vi "Super Market Billing System edit 5.vi"() -> ()   [LabVIEW 2021]
uses:
  <vilib>/Utility/file.llb/Write Delimited Spreadsheet (string).vi
  <vilib>/regexp/Match Regular Expression.xnode
panel:
  in  "Tab Control":T1(tab)
  in  "2":bool caption="Blank Button"
  in  "1":bool caption="Blank Button"
  in  "Address":string
  in  "Telephone No:":string
  in  "Password":string
  in  "Email":string
  in  "Register Now":bool
  out "Horizontal Progress Bar 3":u8(slide) scale=0.0..100.0
  in  "adress":string
  out "Horizontal Progress Bar":u8(slide) scale=0.0..100.0
  in  "password":string
  in  "Email":string
  in  "OK Button":bool
  in  "Rise 5Kg":bool
  in  "Dal 1Kg":bool
  in  "Salt 400g":bool
  in  "Coconut Oil 1L":bool
  in  "Cilli Powder 100g":bool
  in  "Curry Powder 100g":bool
  in  "Turmeric Powder 50g":bool
  in  "Milk Powder 1kg":bool
  in  "Sugar  1kg":bool
  out "Rs.":dbl
  out "Rs.":dbl
  out "Rs.":dbl
  out "Rs.":dbl
  in  "Quantitiy":dbl min=0.0 format="%#.1f"
  out "Rs.":dbl
  in  "Quantitiy":dbl min=0.0 format="%#.1f"
  out "Rs":dbl
  in  "Quantitiy":dbl min=0.0 format="%#.1f"
  out "Rs.":dbl
  in  "Quantitiy":dbl min=0.0 format="%#.1f"
  in  "Quantitiy":dbl min=0.0 format="%#.1f"
  in  "Quantitiy":dbl min=0.0 format="%#.1f"
  in  "Quantitiy":dbl min=0.0 format="%#.1f"
  in  "Quantitiy":dbl min=0.0 format="%#.1f"
  in  "Tea 100g":bool
  in  "Quantitiy":dbl min=0.0 format="%#.1f"
  in  "Quantitiy":dbl min=0.0 format="%#.1f"
  out "Rs.":dbl
  out "Rs.":dbl
  out "Rs.":dbl
  out "Rs.":dbl
  out "Rs.":dbl
  out "Rs.":dbl
  out "Rs.":dbl
  out "Rs. 5":dbl
  out "Rs. 6":dbl
  out "Rs.":dbl
  out "Rs.":dbl
  out "Rs.":dbl
  out "Rs.":dbl
  out "Discount   Rs.":dbl format="%#.2f"
  in  "kg":dbl min=0.0 format="%#.3f"
  in  "Papaya":bool
  in  "kg":dbl min=0.0 format="%#.3f"
  in  "Graps":bool
  in  "kg":dbl min=0.0 format="%#.3f"
  in  "Orange":bool
  in  "kg":dbl min=0.0 format="%#.3f"
  in  "Apple":bool
  in  "kg":dbl min=0.0 format="%#.3f"
  in  "Banana":bool
  out "Bill   Rs.":dbl format="%#.2f"
  out "Discount percentage":string
  out "Total Bill   Rs.":dbl format="%#.2f"
  in  "kg":dbl min=0.0 format="%#.3f"
  in  "Cabege":bool
  in  "kg":dbl min=0.0 format="%#.3f"
  in  "Bringle":bool
  in  "kg":dbl min=0.0 format="%#.3f"
  in  "Beans":bool
  in  "kg":dbl min=0.0 format="%#.3f"
  in  "Leeks":bool
  in  "kg":dbl min=0.0 format="%#.3f"
  in  "Carrot":bool
  in  "stop":bool
  in  "stop 2":bool
  out "Your Bill Details":string
  in  "stop 3":bool
  # "WELCOME TO A SUPER MARCKET...."
  # "Register Here"
  # "Logging Here"
  # "Price per 1kg (Rs.)"
  # "Quantities(kg)"
  # "Price  (Rs.)"
  # "Quantities"
  # "Vegetables"
  # "Product List"
  # "Fruits"
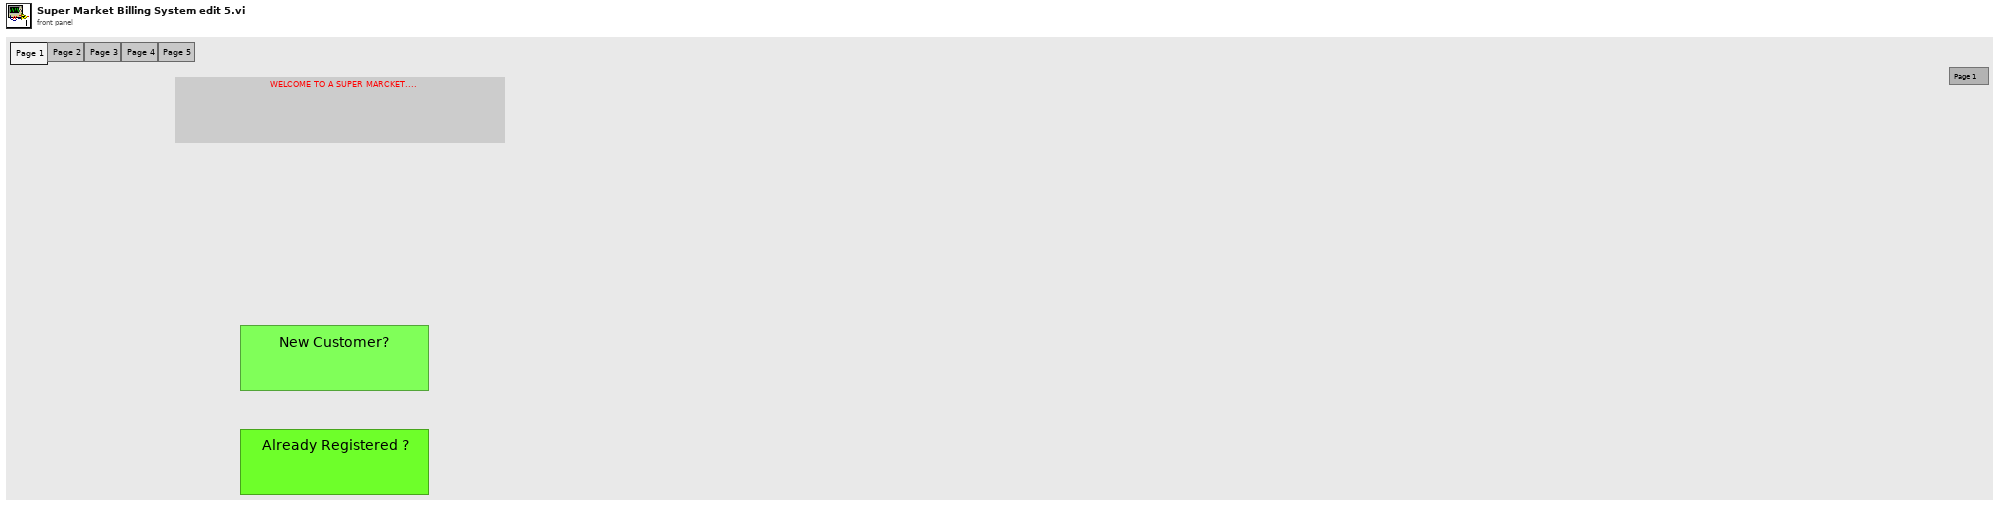
[diagram p1: front panel]
types:
  T1 = enum32{"Page 1", "Page 2", "Page 3", "Page 4", "Page 5"}
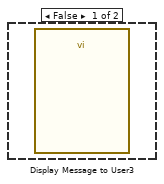
[diagram p2: hidden frame]
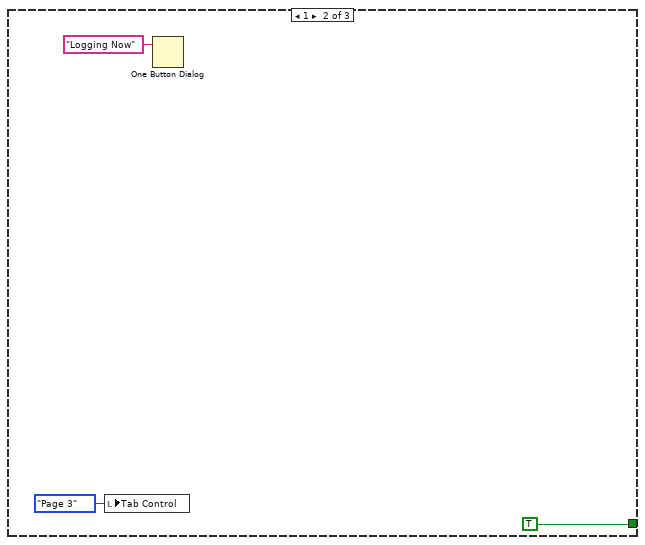
[diagram p4: hidden frame]
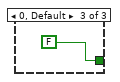
[diagram p5: hidden frame]
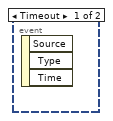
[diagram p6: hidden frame]
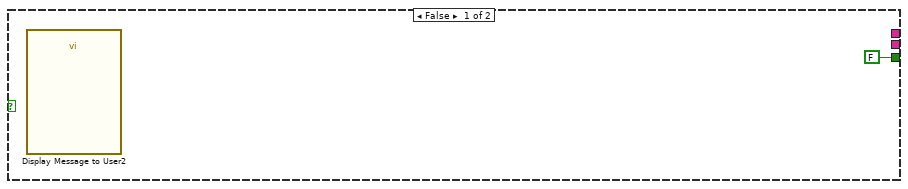
[diagram p7: hidden frame]
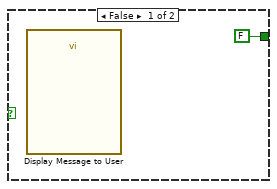
[diagram p8: hidden frame]
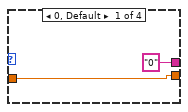
[diagram p9: hidden frame]
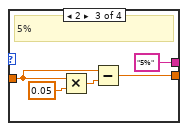
[diagram p10: hidden frame]
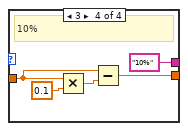
[diagram p11: hidden frame]
diagram:
  n1 = while {
    stop <- FALSE stop-if-true
    n2 = flat-sequence {
      tunnel: [w95] -> w51
      tunnel: [w89] -> w6
      tunnel: w51 -> [w448]
      tunnel: w6 -> [w376]
      frame #0 {
        n3 = while {
          stop <- w53 stop-if-true
          n4 = Build Array("1", "2") -> (w55:bool[])
          n5 = Boolean Array To Number(Boolean array=w55) -> (number=w56:u32)
          n6 = case shown="2" w56 {
            tunnel: [w58 TRUE ("Register Now") FALSE] -> w53
            frame 2 {
              n7 = while {
                tunnel: ["Register Now"] -> w58
                stop <- "Register Now" stop-if-true
                n8 = local write "Tab Control"(T1."Page 2" ("Tab Control")) -> ()
                n9 = case shown="True" "Register Now" {
                  frame False {
                  }
                  frame True {
                    n10 = for {
                      N: 100 -> [_]
                      i -> [w64]
                      n11 = Increment(x=w64) -> (x+1=→"Horizontal Progress Bar 3":i32)
                      n12 = Wait (ms)(milliseconds to wait=u32 50 ("millisecond timer value")) -> ()  [unwired: 1 out]
                    }
                  }
                }
              }
              n13 = case shown="True" w58 {
                frame False {
                  n14 = call "Display Message to User3"() -> ()  [unwired: 10 in, 2 out]
                }
                frame True {
                  n15 = local write "Tab Control"(T1."Page 1" ("Tab Control")) -> ()
                }
              }
            }
            frame 1 {
              n16 = local write "Tab Control"(T1."Page 3" ("Tab Control")) -> ()
              n17 = One Button Dialog(message="Logging Now") -> ()  [unwired: 1 in, 1 out]
            }
            frame 0, Default {
            }
          }
        }
      }
      frame #1 {
        n18 = Build Array("Email  :", "Email") -> (w74:string[])
        n19 = Build Array("Password  :" ("element"), "Password") -> (w73:string[])
        n20 = call-poly <vilib>:"Write Delimited Spreadsheet.vi"("file path (dialog if empty)"=path "E:/1.txt", "2D data"=string[][] [["A", ""], ["B", ""], ["C", ""], ["D", ""], ["E", ""], ["F", ""]]) -> ("new file path (Not A Path if cancelled)"=w75:path)  [unwired: 12 in, 1 out]
        n21 = while {
          shift-right: [w85] -> _
          shift-left: 0 -> [w86]
          tunnel: w75 -> [w84]
          tunnel: w74 -> [w83]
          tunnel: w73 -> [w82]
          stop <- FALSE stop-if-true
          n22 = Increment(x=w86) -> (x+1=w85:i32)
          n23 = Insert Into Array(array=w83, new element=w82) -> (w81:string[])  [unwired: 1 in]
          n24 = call-poly <vilib>:"Write Delimited Spreadsheet.vi"("file path (dialog if empty)"=w84, "1D data"=w81) -> ()  [unwired: 12 in, 2 out]
        }
      }
      frame #2 {
        n25 = while {
          tunnel: [w101] -> w91
          tunnel: [w100] -> w90
          stop <- w99 stop-if-true
          n26 = event shown="[1] \"OK Button\": Value Change" {
            selector: _ -> [_ _]
            dyn-events: _ -> [_ _]
            timeout: _ -> [_ _]
            tunnel: [_ "OK Button"] -> w98
            event Timeout {
              n27 = event-data() -> ()  [unwired: 1 in, 3 out]
            }
            event "OK Button": Value Change {
              n28 = event-data() -> ()  [unwired: 1 in, 6 out]
            }
          }
          n29 = case shown="True" w98 {
            tunnel: [_ w107] -> w101
            tunnel: [_ w108] -> w100
            tunnel: [FALSE w106] -> w99
            frame False {
              n30 = call "Display Message to User2"() -> ()  [unwired: 10 in, 2 out]
            }
            frame True {
              n31 = Read from Text File(file (use dialog)=path "E:/new 1.txt") -> (text=w110:string)  [unwired: 3 in, 3 out]
              n32 = while {
                tunnel: w110 -> [w130]
                tunnel: ["adress"] -> w107
                tunnel: ["Email"] -> w108
                tunnel: [w117] -> w105
                stop <- w117 stop-if-true
                n33 = feedback #1(w130) -> (w129:string)
                n34 = xnode "Match Regular Expression"("input string"=w129, "regular expression"="\n") -> ("before match"=w126:string, "after match"=w128:string)  [unwired: 4 in, 3 out]
                n35 = feedback-in #1(w128) -> ()
                n36 = xnode "Match Regular Expression"("input string"=w126, "regular expression"=",") -> ("before match"=w123:string, "after match"=w124:string)  [unwired: 4 in, 3 out]
                n37 = Equal?(x="Email", y=w123) -> (x = y?=w121:bool)
                n38 = Equal?(x=w124, y="password") -> (x = y?=w120:bool)
                n39 = And(x=w121, y=w120) -> (x .and. y?=w117:bool)
              }
              n40 = local write "Tab Control"(T1."Page 3" ("Tab Control")) -> ()
              n41 = case shown="True" w105 {
                tunnel: [FALSE TRUE] -> w106
                frame False {
                  n42 = call "Display Message to User"() -> ()  [unwired: 10 in, 2 out]
                }
                frame True {
                  n43 = for {
                    N: 100 -> [_]
                    i -> [w114]
                    n44 = Increment(x=w114) -> (x+1=→"Horizontal Progress Bar":i32)
                    n45 = Wait (ms)(milliseconds to wait=u32 50 ("millisecond timer value")) -> ()  [unwired: 1 out]
                  }
                }
              }
            }
          }
        }
        n46 = Get Date/Time In Seconds() -> (seconds since 1Jan1904=w96:timestamp)
        n47 = Get Date/Time String(seconds (now)=w96) -> (date string=w94:string, time string=w97:string)  [unwired: 2 in]
        n48 = Build Array("Odered Date  :" ("element"), w94, "       Odered Time  :" ("element"), w97) -> (w95:string[])
        n49 = Build Array("Address  :" ("element"), w91, "              User Name  :" ("element"), w90) -> (w89:string[])
      }
      frame #3 {
        n50 = while {
          tunnel: [w618] -> w440
          tunnel: [w615] -> w442
          tunnel: [w614] -> w443
          tunnel: [w605] -> w406
          tunnel: [w585] -> w404
          tunnel: [w584] -> w402
          tunnel: [w575] -> w400
          tunnel: [w574] -> w398
          tunnel: [w573] -> w396
          tunnel: [w572] -> w394
          tunnel: [w571] -> w392
          tunnel: [w570] -> w390
          tunnel: [w569] -> w388
          tunnel: ["kg"] -> w447
          tunnel: ["kg"] -> w446
          tunnel: [w565] -> w401
          tunnel: [w563] -> w399
          tunnel: [w560] -> w397
          tunnel: [w559] -> w395
          tunnel: [w558] -> w393
          tunnel: [w555] -> w391
          tunnel: [w552] -> w389
          tunnel: [w551] -> w387
          tunnel: [w520] -> w439
          tunnel: [w519] -> w437
          tunnel: [w518] -> w435
          tunnel: [w517] -> w434
          tunnel: [w516] -> w432
          tunnel: [w515] -> w430
          tunnel: [w514] -> w423
          tunnel: [w513] -> w427
          tunnel: [w512] -> w425
          tunnel: [w511] -> w424
          tunnel: [w508] -> w436
          tunnel: [w507] -> w438
          tunnel: [w505] -> w421
          tunnel: [w503] -> w433
          tunnel: [w501] -> w431
          tunnel: [w496] -> w429
          tunnel: [w495] -> w428
          tunnel: [w494] -> w426
          tunnel: [w493] -> w422
          tunnel: ["Total Bill                                                                          Rs." ("element")] -> w365
          stop <- "stop" stop-if-true
          w631 = 200.0 ("price")
          w628 = 430.0 ("price")
          w625 = 250.0 ("price")
          w622 = 230.0 ("price")
          w619 = 150.0 ("price")
          w646 = 600.0 ("price")
          w643 = 280.0 ("price")
          w640 = 540.0 ("price")
          w637 = 780.0 ("price")
          w634 = 1000.0 ("price")
          w684 = 150.0 ("price")
          w681 = 700.0 ("price")
          w678 = 2000.0 ("price")
          w675 = 180.0 ("price")
          w672 = 150.0  # price
          w697 = 190.0 ("price")
          w694 = 800.0 ("price")
          w691 = 260.0 ("price")
          w689 = 500.0 ("price")
          w686 = 1050.0 ("price")
          n51 = Wait (ms)(milliseconds to wait=u32 500) -> ()  [unwired: 1 out]
          n52 = Boolean To (0,1)(Boolean="Sugar  1kg") -> (0, 1=w682:i16)
          n53 = Boolean To (0,1)(Boolean="Curry Powder 100g") -> (0, 1=w671:i16)
          n54 = Boolean To (0,1)(Boolean="Turmeric Powder 50g") -> (0, 1=w676:i16)
          n55 = Boolean To (0,1)(Boolean="Milk Powder 1kg") -> (0, 1=w677:i16)
          n56 = Boolean To (0,1)(Boolean="Tea 100g") -> (0, 1=w683:i16)
          n57 = Boolean To (0,1)(Boolean="Rise 5Kg") -> (0, 1=w613:i16)
          n58 = Boolean To (0,1)(Boolean="Dal 1Kg") -> (0, 1=w611:i16)
          n59 = Boolean To (0,1)(Boolean="Salt 400g") -> (0, 1=w690:i16)
          n60 = Boolean To (0,1)(Boolean="Coconut Oil 1L") -> (0, 1=w696:i16)
          n61 = Boolean To (0,1)(Boolean="Cilli Powder 100g") -> (0, 1=w612:i16)
          n62 = Boolean To (0,1)(Boolean="Banana") -> (0, 1=w609:i16)
          n63 = Boolean To (0,1)(Boolean="Apple") -> (0, 1=w623:i16)
          n64 = Boolean To (0,1)(Boolean="Orange") -> (0, 1=w624:i16)
          n65 = Boolean To (0,1)(Boolean="Graps") -> (0, 1=w629:i16)
          n66 = Boolean To (0,1)(Boolean="Papaya") -> (0, 1=w630:i16)
          n67 = Boolean To (0,1)(Boolean="Carrot") -> (0, 1=w633:i16)
          n68 = Boolean To (0,1)(Boolean="Leeks") -> (0, 1=w638:i16)
          n69 = Boolean To (0,1)(Boolean="Beans") -> (0, 1=w639:i16)
          n70 = Boolean To (0,1)(Boolean="Bringle") -> (0, 1=w644:i16)
          n71 = Boolean To (0,1)(Boolean="Cabege") -> (0, 1=w645:i16)
          n72 = Multiply(x=w682, y="Quantitiy") -> (x*y=w680:dbl)
          n73 = Multiply(x=w671, y="Quantitiy") -> (x*y=w673:dbl)
          n74 = Multiply(x=w676, y="Quantitiy") -> (x*y=w674:dbl)
          n75 = Multiply(x=w677, y="Quantitiy") -> (x*y=w679:dbl)
          n76 = Multiply(x=w683, y="Quantitiy") -> (x*y=w685:dbl)
          n77 = Multiply(x=w613, y="Quantitiy") -> (x*y=w687:dbl)
          n78 = Multiply(x=w611, y="Quantitiy") -> (x*y=w688:dbl)
          n79 = Multiply(x=w690, y="Quantitiy") -> (x*y=w692:dbl)
          n80 = Multiply(x=w696, y="Quantitiy") -> (x*y=w693:dbl)
          n81 = Multiply(x=w612, y="Quantitiy") -> (x*y=w698:dbl)
          n82 = Multiply(x=w609, y="kg") -> (x*y=w620:dbl)
          n83 = Multiply(x=w623, y="kg") -> (x*y=w621:dbl)
          n84 = Multiply(x=w624, y="kg") -> (x*y=w626:dbl)
          n85 = Multiply(x=w629, y="kg") -> (x*y=w627:dbl)
          n86 = Multiply(x=w630, y="kg") -> (x*y=w632:dbl)
          n87 = Multiply(x=w633, y="kg") -> (x*y=w635:dbl)
          n88 = Multiply(x=w638, y="kg") -> (x*y=w636:dbl)
          n89 = Multiply(x=w639, y="kg") -> (x*y=w641:dbl)
          n90 = Multiply(x=w644, y="kg") -> (x*y=w642:dbl)
          n91 = Multiply(x=w645, y="kg") -> (x*y=w647:dbl)
          n92 = Multiply(x=w681, y=w680) -> (x*y=w482:dbl)
          n93 = Multiply(x=w672, y=w673) -> (x*y=w483:dbl)
          n94 = Multiply(x=w675, y=w674) -> (x*y=w484:dbl)
          n95 = Multiply(x=w678, y=w679) -> (x*y=w485:dbl)
          n96 = Multiply(x=w684, y=w685) -> (x*y=w487:dbl)
          n97 = Multiply(x=w686, y=w687) -> (x*y=w488:dbl)
          n98 = Multiply(x=w689, y=w688) -> (x*y=w486:dbl)
          n99 = Multiply(x=w691, y=w692) -> (x*y=w489:dbl)
          n100 = Multiply(x=w694, y=w693) -> (x*y=w490:dbl)
          n101 = Multiply(x=w697, y=w698) -> (x*y=w491:dbl)
          n102 = Multiply(x=w619, y=w620) -> (x*y=w610:dbl)
          n103 = Multiply(x=w622, y=w621) -> (x*y=w662:dbl)
          n104 = Multiply(x=w625, y=w626) -> (x*y=w663:dbl)
          n105 = Multiply(x=w628, y=w627) -> (x*y=w664:dbl)
          n106 = Multiply(x=w631, y=w632) -> (x*y=w665:dbl)
          n107 = Multiply(x=w634, y=w635) -> (x*y=w666:dbl)
          n108 = Multiply(x=w637, y=w636) -> (x*y=w667:dbl)
          n109 = Multiply(x=w640, y=w641) -> (x*y=w668:dbl)
          n110 = Multiply(x=w643, y=w642) -> (x*y=w669:dbl)
          n111 = Multiply(x=w646, y=w647) -> (x*y=w670:dbl)
          n112 = Compound Arithmetic op=ADD(w482, w483, w484, w485, w487, w488, w486, w489, w490, w491, w610, w662, w663, w664, w665, w666, w667, w668, w669, w670) -> (w481:dbl)
          "Bill   Rs." <- w481
          n113 = Greater?(x=w481, y=5000.0) -> (0:w659:bool)
          n114 = Greater?(x=w481, y=20000.0) -> (0:w661:bool)
          n115 = Greater?(x=w481, y=10000.0) -> (0:w660:bool)
          n116 = Select(t=1.0, s=w659, f=0.0) -> (s? t:f=w655:dbl)
          n117 = Select(t=2.0, s=w660, f=w655) -> (s? t:f=w656:dbl)
          n118 = Select(t=3.0, s=w661, f=w656) -> (s? t:f=w657:dbl)
          n119 = case shown="1" w657 {
            tunnel: [w701 w705 w708 w713] -> w617
            tunnel: w481 -> [w701 w704 w709 w714]
            tunnel: ["0" ("discount") "2%" ("discount") "5%" ("discount") "10%" ("discount")] -> w658
            frame 0, Default {
            }
            frame 1 {
              # "2%"
              n120 = Multiply(x=w704, y=0.02) -> (x*y=w702:dbl)
              n121 = Subtract(x=w704, y=w702) -> (x-y=w705:dbl)
            }
            frame 2 {
              # "5%"
              n122 = Multiply(x=w709, y=0.05) -> (x*y=w710:dbl)
              n123 = Subtract(x=w709, y=w710) -> (x-y=w708:dbl)
            }
            frame 3 {
              # "10%"
              n124 = Multiply(x=w714, y=0.1) -> (x*y=w715:dbl)
              n125 = Subtract(x=w714, y=w715) -> (x-y=w713:dbl)
            }
          }
          "Total Bill   Rs." <- w617
          "Discount percentage" <- w658
          n126 = Subtract(x=w481, y=w617) -> (x-y=w616:dbl)
          "Discount   Rs." <- w616
          n127 = Number To Fractional String(number=w481) -> (F-format string=w618:string)  [unwired: 3 in]
          n128 = Number To Fractional String(number=w616) -> (F-format string=w614:string)  [unwired: 3 in]
          n129 = Number To Fractional String(number=w617) -> (F-format string=w615:string)  [unwired: 3 in]
          n130 = Select(t="Leeks                                                       ", s="Leeks", f="Leeks                                                      ") -> (s? t:f=w572:string)
          n131 = Select(t="Graps                                                      " ("f"), s="Graps", f="Graps                                                       ") -> (s? t:f=w575:string)
          n132 = Select(t="Apple                                                      ", s="Apple", f="Apple                                                      ") -> (s? t:f=w585:string)
          n133 = Select(t="Beans                                                       ", s="Beans", f="Beans                                                      ") -> (s? t:f=w571:string)
          n134 = Number To Fractional String(number="Quantitiy") -> (F-format string=w507:string)  [unwired: 3 in]
          n135 = Number To Fractional String(number="Quantitiy") -> (F-format string=w508:string)  [unwired: 3 in]
          n136 = Number To Fractional String(number="Quantitiy") -> (F-format string=w493:string)  [unwired: 3 in]
          n137 = Number To Fractional String(number="Quantitiy") -> (F-format string=w503:string)  [unwired: 3 in]
          n138 = Number To Fractional String(number="Quantitiy") -> (F-format string=w501:string)  [unwired: 3 in]
          n139 = Number To Fractional String(number="Quantitiy") -> (F-format string=w505:string)  [unwired: 3 in]
          n140 = Number To Fractional String(number="Quantitiy") -> (F-format string=w496:string)  [unwired: 3 in]
          n141 = Number To Fractional String(number="Quantitiy") -> (F-format string=w495:string)  [unwired: 3 in]
          n142 = Number To Fractional String(number="Quantitiy") -> (F-format string=w494:string)  [unwired: 3 in]
          n143 = Number To Fractional String(number="kg") -> (F-format string=w551:string)  [unwired: 3 in]
          n144 = Number To Fractional String(number="kg") -> (F-format string=w565:string)  [unwired: 3 in]
          n145 = Number To Fractional String(number="kg") -> (F-format string=w563:string)  [unwired: 3 in]
          n146 = Number To Fractional String(number="kg") -> (F-format string=w560:string)  [unwired: 3 in]
          n147 = Number To Fractional String(number="kg") -> (F-format string=w559:string)  [unwired: 3 in]
          n148 = Number To Fractional String(number="kg") -> (F-format string=w558:string)  [unwired: 3 in]
          n149 = Number To Fractional String(number="kg") -> (F-format string=w555:string)  [unwired: 3 in]
          n150 = Number To Fractional String(number="kg") -> (F-format string=w552:string)  [unwired: 3 in]
          n151 = Select(t="Suger 1kg                                               ", s="Sugar  1kg", f="Suger 1kg                                               ") -> (s? t:f=w520:string)
          n152 = Select(t="Curry Powder 100g                                        ", s="Curry Powder 100g", f="Curry Powder 100g                                        ") -> (s? t:f=w519:string)
          n153 = Select(t="Dal 1Kg                                                     ", s="Dal 1Kg", f="Dal 1Kg                                                     ") -> (s? t:f=w511:string)
          n154 = Select(t="Turmeric Powder 50g                              ", s="Turmeric Powder 50g", f="Turmeric Powder 50g                              ") -> (s? t:f=w518:string)
          n155 = Select(t="Milk Powder 1kg                                      ", s="Milk Powder 1kg", f="Milk Powder 1kg                                      ") -> (s? t:f=w517:string)
          n156 = Select(t="Tea 100g                                                     ", s="Tea 100g", f="Tea 100g                                                      ") -> (s? t:f=w516:string)
          n157 = Select(t="Salt 400g                                                            ", s="Salt 400g", f="Salt 400g                                                            ") -> (s? t:f=w515:string)
          n158 = Select(t="Coconut Oil 1L                                         ", s="Coconut Oil 1L", f="Coconut Oil 1L                                               ") -> (s? t:f=w514:string)
          n159 = Select(t="Cilli Powder 100g                                              ", s="Cilli Powder 100g", f="Cilli Powder 100g                                             ") -> (s? t:f=w513:string)
          n160 = Select(t="Rise 5Kg                                                  ", s="Rise 5Kg", f="Rise 5Kg                                                 ") -> (s? t:f=w512:string)
          n161 = Select(t="Cabege                                                ", s="Cabege", f="Cabege                                                 ") -> (s? t:f=w569:string)
          n162 = Select(t="Banana                                                  ", s="Banana", f="Banana                                                   ") -> (s? t:f=w605:string)
          n163 = Select(t="Orange                                                   ", s="Orange", f="Orange                                                    ") -> (s? t:f=w584:string)
          n164 = Select(t="Papaya                                                    ", s="Papaya", f="Papaya                                                    ") -> (s? t:f=w574:string)
          n165 = Select(t="Carrot                                                      ", s="Carrot", f="Carrot                                                       ") -> (s? t:f=w573:string)
          n166 = Select(t="Bringle                                                      ", s="Bringle", f="Bringle                                                      ") -> (s? t:f=w570:string)
          "Rs." <- w686
          "Rs." <- w689
          "Rs." <- w691
          "Rs." <- w694
          "Rs." <- w697
          "Rs." <- w672
          "Rs." <- w675
          "Rs." <- w678
          "Rs" <- w681
          "Rs." <- w684
          "Rs." <- w634
          "Rs." <- w637
          "Rs." <- w640
          "Rs." <- w643
          "Rs. 6" <- w646
          "Rs. 5" <- w619
          "Rs." <- w622
          "Rs." <- w625
          "Rs." <- w628
          "Rs." <- w631
        }
        n167 = Build Array(w439, w438) -> (w416:string[])
        n168 = Build Array(w437, w436) -> (w415:string[])
        n169 = Build Array(w424, w422) -> (w407:string[])
        n170 = Build Array(w435, w421) -> (w414:string[])
        n171 = Build Array(w434, w433) -> (w413:string[])
        n172 = Build Array(w432, w431) -> (w412:string[])
        n173 = Build Array(w430, w429) -> (w411:string[])
        n174 = Build Array(w423, w428) -> (w410:string[])
        n175 = Build Array(w427, w426) -> (w409:string[])
        n176 = Build Array(w425, w421) -> (w408:string[])
        n177 = Build Array(w388, w387) -> (w377:string[])
        n178 = Build Array(w402, w401) -> (w384:string[])
        n179 = Build Array(w400, w399) -> (w383:string[])
        n180 = Build Array(w398, w397) -> (w382:string[])
        n181 = Build Array(w396, w395) -> (w381:string[])
        n182 = Build Array(w394, w393) -> (w380:string[])
        n183 = Build Array(w392, w391) -> (w379:string[])
        n184 = Build Array(w390, w389) -> (w378:string[])
        n185 = Build Array("Dicount                                                                          Rs." ("element"), w443) -> (w418:string[])
        n186 = Build Array(w365, w442) -> (w417:string[])
        n187 = Number To Fractional String(number=w447) -> (F-format string=w405:string)  [unwired: 3 in]
        n188 = Number To Fractional String(number=w446) -> (F-format string=w403:string)  [unwired: 3 in]
        n189 = Build Array("                            ", "                    " ("element")) -> (w371:string[])
        n190 = call-poly <vilib>:"Write Delimited Spreadsheet.vi"("2D data"=string[][] [["Email    "], ["Address "], ["Odered date"], ["Time"], ["A"], ["B "], ["C    "], ["D    "], ["E   "], [" F   "], ["G    "], [" H   "], [" I   "], ["   j "], ["   k "], ["   l "], ["   m "], ["   n "], ["   o "], ["    p"], ["   q "], ["   r "], ["   s "], ["   t "], ["   u "], ["   v "], ["   w "], ["   x "], ["   y "], ["   z "]] ("delimiter (\\t)")) -> ("new file path (Not A Path if cancelled)"=w444:path)  [unwired: 13 in, 1 out]
        n191 = Build Array(w448) -> (w420:string[][])
        n192 = Build Array(w376) -> (w375:string[][])
        n193 = Build Array(w406, w405) -> (w386:string[])
        n194 = Build Array(w404, w403) -> (w385:string[])
        n195 = Build Array("Bill                                                                                   Rs." ("element"), w440) -> (w419:string[])
        n196 = local write "Tab Control"(T1."Page 4" ("Tab Control")) -> ()
        n197 = Build Array("                                                          " ("element"), "Quantity" ("element")) -> (w368:string[])
        n198 = while {
          tunnel: w444 -> [w479]
          shift-right: [w476] -> _
          shift-left: 0 -> [w477]
          tunnel: w420 -> [w475]
          tunnel: w419 -> [w470]
          tunnel: w418 -> [w471]
          tunnel: w417 -> [w472]
          tunnel: w416 -> [_]
          tunnel: w415 -> [w451]
          tunnel: w414 -> [w453]
          tunnel: w413 -> [w454]
          tunnel: w412 -> [w455]
          tunnel: w411 -> [w456]
          tunnel: w410 -> [w457]
          tunnel: w409 -> [w458]
          tunnel: w408 -> [w459]
          tunnel: w407 -> [w452]
          tunnel: w386 -> [w461]
          tunnel: w385 -> [w462]
          tunnel: w384 -> [w463]
          tunnel: w383 -> [w464]
          tunnel: w382 -> [w465]
          tunnel: w381 -> [w466]
          tunnel: w380 -> [w467]
          tunnel: w379 -> [w468]
          tunnel: w378 -> [w469]
          tunnel: w377 -> [w460]
          tunnel: w375 -> [w473]
          tunnel: w371 -> [w450]
          tunnel: w368 -> [w449]
          stop <- "stop 2" stop-if-true
          n199 = Insert Into Array "Insert Into Array"(array=w475, new element #1=w473, new element #2=w450, new element #3=w449, new element #4=w451, new element #5=w452, new element #6=w452, new element #7=w453, new element #8=w454, new element #9=w455, new element #10=w456, new element #11=w457, new element #12=w458, new element #13=w459, new element #14=w460, new element #15=w461, new element #16=w462, new element #17=w463, new element #18=w464, new element #19=w465, new element #20=w466, new element #21=w467, new element #22=w468, new element #23=w469, new element #24=w470, new element #25=w471, new element #26=w472) -> (w474:string[][])  [unwired: 2 in]
          n200 = Increment(x=w477) -> (x+1=w476:i32)
          n201 = call-poly <vilib>:"Write Delimited Spreadsheet.vi"("file path (dialog if empty)"=w479, "2D data"=w474) -> ()  [unwired: 12 in, 2 out]
        }
      }
      frame #4 {
        n202 = while {
          stop <- "stop 3" stop-if-true
          n203 = Read from Text File(file (use dialog)=path "E:/2.txt") -> (text=→"Your Bill Details":string)  [unwired: 3 in, 3 out]
        }
        n204 = local write "Tab Control"(T1."Page 5" ("Tab Control")) -> ()
      }
      frame #5 {
        n205 = local write "Tab Control"(T1."Page 1" ("Tab Control")) -> ()
      }
    }
    n206 = local write "Email"("" ("Email")) -> ()
    n207 = local write "Password"("" ("Password")) -> ()
    n208 = local write "kg"(0.0 ("kg")) -> ()
    n209 = local write "kg"(0.0 ("kg")) -> ()
    n210 = local write "Discount   Rs."(0.0 ("Discount   Rs.")) -> ()
    n211 = local write "Salt 400g"(FALSE ("Salt 400g")) -> ()
    n212 = local write "adress"("" ("adress")) -> ()
    n213 = local write "password"("" ("String 2")) -> ()
    n214 = local write "Graps"(FALSE ("Graps")) -> ()
    n215 = local write "Cabege"(FALSE ("Cabege")) -> ()
    n216 = local write "Quantitiy"(0.0 ("quantity 16")) -> ()
    n217 = local write "Apple"(FALSE ("Apple")) -> ()
    n218 = local write "Email"("" ("String")) -> ()
    n219 = local write "Papaya"(FALSE ("Papaya")) -> ()
    n220 = local write "kg"(0.0 ("kg")) -> ()
    n221 = local write "kg"(0.0 ("kg")) -> ()
    n222 = local write "Quantitiy"(0.0 ("quantity 11")) -> ()
    n223 = local write "Dal 1Kg"(FALSE ("Dal 1Kg")) -> ()
    n224 = local write "Milk Powder 1kg"(FALSE ("Milk Powder 1kg")) -> ()
    n225 = local write "Bringle"(FALSE ("Bringle")) -> ()
    n226 = local write "Banana"(FALSE ("Banana")) -> ()
    n227 = local write "Sugar  1kg"(FALSE ("Sugar  1kg")) -> ()
    n228 = local write "kg"(0.0 ("kg")) -> ()
    n229 = local write "Cilli Powder 100g"(FALSE ("Cilli Powder 100g")) -> ()
    n230 = local write "Tea 100g"(FALSE ("Tea 100g")) -> ()
    n231 = local write "Quantitiy"(0.0 ("Quantities")) -> ()
    n232 = local write "Quantitiy"(0.0 ("Quantities 4")) -> ()
    n233 = local write "kg"(0.0 ("kg")) -> ()
    n234 = local write "Rise 5Kg"(FALSE ("Rise 5Kg")) -> ()
    n235 = local write "Beans"(FALSE ("Beans")) -> ()
    n236 = local write "Coconut Oil 1L"(FALSE ("Coconut Oil 1L")) -> ()
    n237 = local write "Turmeric Powder 50g"(FALSE ("Turmeric Powder 50g")) -> ()
    n238 = local write "kg"(0.0 ("kg")) -> ()
    n239 = local write "Carrot"(FALSE ("Carrot")) -> ()
    n240 = local write "Curry Powder 100g"(FALSE ("Curry Powder 100g")) -> ()
    n241 = local write "Leeks"(FALSE ("Leeks")) -> ()
    n242 = local write "Discount percentage"("0" ("Discount percentage")) -> ()
    n243 = local write "Bill   Rs."(0.0 ("Bill   Rs.")) -> ()
    n244 = local write "Total Bill   Rs."(0.0 ("Total Bill   Rs.")) -> ()
    n245 = local write "kg"(0.0 ("kg")) -> ()
    n246 = local write "Orange"(FALSE ("Orange")) -> ()
    n247 = local write "kg"(0.0 ("kg")) -> ()
    n248 = local write "kg"(0.0 ("kg")) -> ()
    n249 = local write "Quantitiy"(0.0 ("quantity 14")) -> ()
    n250 = local write "Quantitiy"(0.0 ("quantity 12")) -> ()
    n251 = local write "Quantitiy"(0.0 ("quantity 10")) -> ()
    n252 = local write "Quantitiy"(0.0 ("quantity 17")) -> ()
    n253 = local write "Quantitiy"(0.0 ("quantity 15")) -> ()
    n254 = local write "Quantitiy"(0.0 ("quantity 13")) -> ()
  }
